vi "Get Config Ref.vi"(8 "error in (no error)":errorcluster, 11 "Configuration In":refnum<class "Configuration.lvclass">) -> (0 "error out":errorcluster, 2 "Reference":variant, 3 "Configuration Out":refnum<class "Configuration.lvclass">)   [LabVIEW 2020, in "Configuration.lvclass"]
doc: "For the configuration interface to work, the class implementing the interface needs to save the reference to the configuration resource in the class attributes. This is an accessor for that attribute which must be implemented by the class."
uses:
  Configuration.lvclass
  Base/Base.lvclass
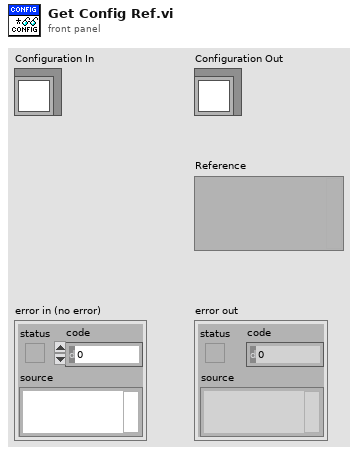
[diagram p1: front panel]
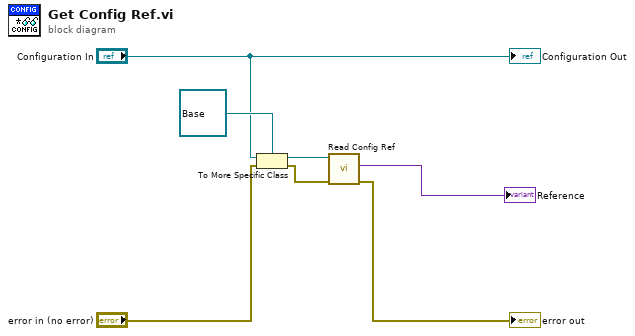
[diagram p0: block diagram]
diagram:
  n1 = To More Specific Class(target class=refnum<class "Base.lvclass"> refnum ("Base.lvclass"), reference="Configuration In", error in="error in (no error)") -> (specific class reference=w5:refnum<class "Base.lvclass">, error out=w3:errorcluster)
  n2 = call "Read Config Ref.vi"("error in (no error)"=w3, "Base In"=w5) -> ("error out"=→"error out":errorcluster, "Config File Refnum"=→"Reference":variant)  [unwired: 7 in, 1 out]
  "Configuration Out" <- "Configuration In"
